vi "setUp.vi"(8 "error in (no error)":errorcluster, 11 "reference in":refnum<class "Test TCP Stream Listener Connect.lvclass">) -> (0 "error out":errorcluster, 3 "reference out":refnum<class "Test TCP Stream Listener Connect.lvclass">)   [LabVIEW 2020, in "Test TCP Stream Listener Connect.lvclass"]
doc: "setUp runs prior to the test method during test execution. Use this method to initialize any object data required by your tests."
uses:
  Test TCP Stream Listener Connect.lvclass
  <vilib>/addons/_JKI Toolkits/VI Tester/TestCase.llb/TestCase.lvclass
  Source/Protocols/TCP Strategy/TCP Stream Listener/TCP Stream Listener.lvclass
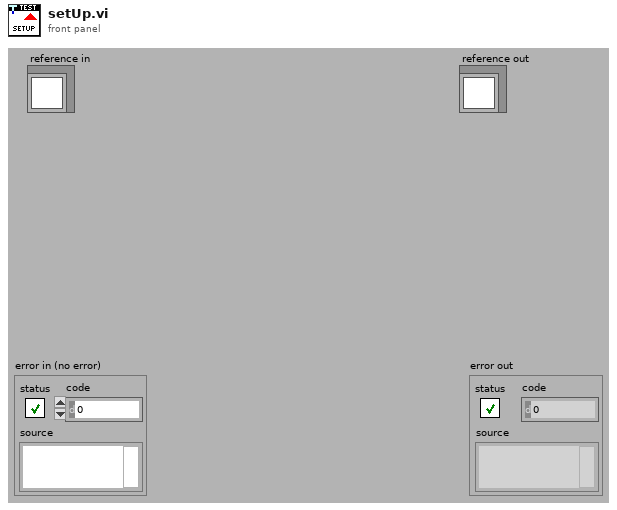
[diagram p1: front panel]
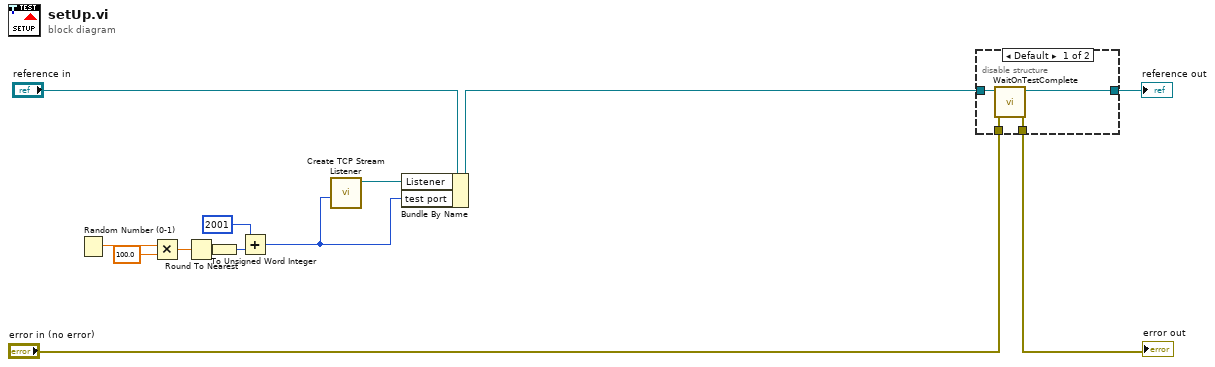
[diagram p0: block diagram]
diagram:
  n1 = Random Number (0-1)() -> (number: 0 to 1=w8:dbl)
  n2 = Multiply(x=w8, y=100.0) -> (x*y=w6:dbl)
  n3 = Round To Nearest(number=w6) -> (nearest integer value=w5:dbl)
  n4 = To Unsigned Word Integer(number=w5) -> (unsigned 16bit integer=w3:u16)
  n5 = Add(x=u16 2001 ("Port"), y=w3) -> (x+y=w1:u16)
  n6 = call "Create TCP Stream Listener.vi"("Local Port"=w1) -> ("TCP Stream Listener"=w2:refnum<class "TCP Stream Listener.lvclass">)  [unwired: 10 in]
  n7 = Bundle By Name(cluster="reference in", "Listener"=w2, "test port"=w1) -> (w9:refnum<class "Test TCP Stream Listener Connect.lvclass">)
  n8 = disable-structure shown="Default" {
    disable-tunnel: "error in (no error)" -> [w17 w18]
    disable-tunnel: [w16 w18] -> w12
    disable-tunnel: [w15 w19] -> w10
    disable-tunnel: w9 -> [w14 w19]
    frame condition #0 (active) {
      n9 = call <vilib>:"WaitOnTestComplete.vi"("error in (no error)"=w17, "TestCase in"=w14) -> ("error out"=w16:errorcluster, "TestCase out"=w15:refnum<class "Test TCP Stream Listener Connect.lvclass">)  [unwired: 8 in]
    }
    frame condition #1 {
    }
  }
  "error out" <- w12
  "reference out" <- w10
